vi "GT Get Di Config.vi"(7 "pDi":T1, 8 "error in (no error)":errorcluster caption="错误输入（无错误）", 9 "diIndex":i16, 10 "diType":i16, 11 "cardNum":i16) -> (0 "error out":errorcluster caption="错误输出", 3 "function return":i16, 5 "pDi out":T1)   [LabVIEW 2020, in "gts1.lvlib"]
doc: "GT_API GT_GetDiConfig(short cardNum,short diType,short diIndex,TDiConfig *pDi);"
uses:
  gts1.lvlib
  dll/32bit/multi_card/gts.dll
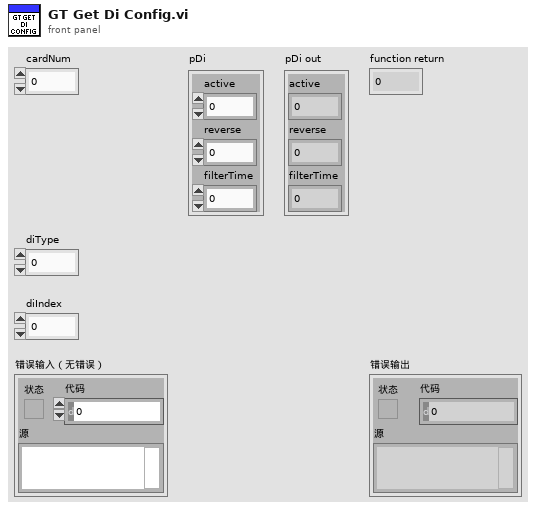
[diagram p1: front panel]
types:
  T1 = cluster{"active":i16, "reverse":i16, "filterTime":i16}
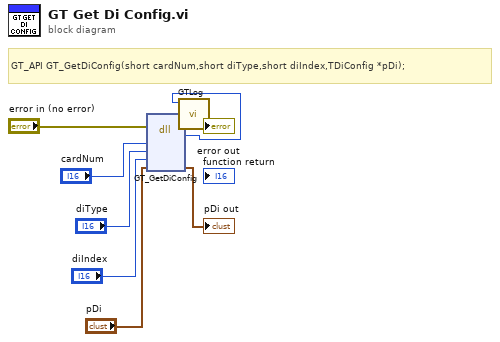
[diagram p0: block diagram]
diagram:
  # "GT_API GT_GetDiConfig(short cardNum,short diType,short diIndex,TDiConfig *pDi);"
  n1 = dll-call lib="C:/1228/dll/32bit/multi_card/gts.dll" fn="GT_GetDiConfig"(error in="error in (no error)", "cardNum"="cardNum", "diType"="diType", "diIndex"="diIndex", "pDi"="pDi") -> (error out=w3:errorcluster, w1:i16, "pDi"=→"pDi out":T1)  [unwired: 5 in, 1 out]
  n2 = call "GTLog.vi"("error in (no error)"=w3, "Numeric"=w1) -> ("error out"=→"error out":errorcluster)  [unwired: 9 in]
